vi "Parse Navigation Results.vi"(9 "Cycle Time":dbl, 10 "Targeting Data In":T1, 11 "Target Data":string) -> (2 "Targeting Data Out":T1)   [LabVIEW 2017, in "VisionHW.lvlib"]
uses:
  VisionHW.lvlib
  TypeDef/CLUST_Targeting Data.ctl
  TypeDef/CLUST_Cube Data.ctl
  TypeDef/CLUST_Road Navigation Data.ctl
  <vilib>/regexp/Match Regular Expression.xnode
panel:
  out "after substring":string
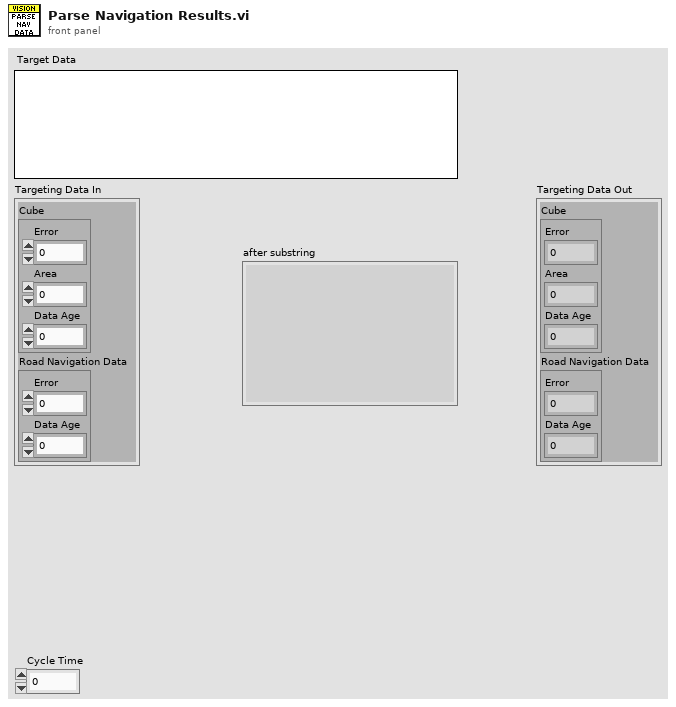
[diagram p1: front panel]
types:
  T1 = typedef "VisionHW.lvlib/CLUST_Targeting Data.ctl" = cluster{"Cube ":T2, "Road Navigation Data":T3}
  T2 = typedef "VisionHW.lvlib/CLUST_Cube Data.ctl" = cluster{"Error":dbl, "Area":dbl, "Data Age":dbl}
  T3 = typedef "VisionHW.lvlib/CLUST_Road Navigation Data.ctl" = cluster{"Error":i32, "Data Age":dbl}
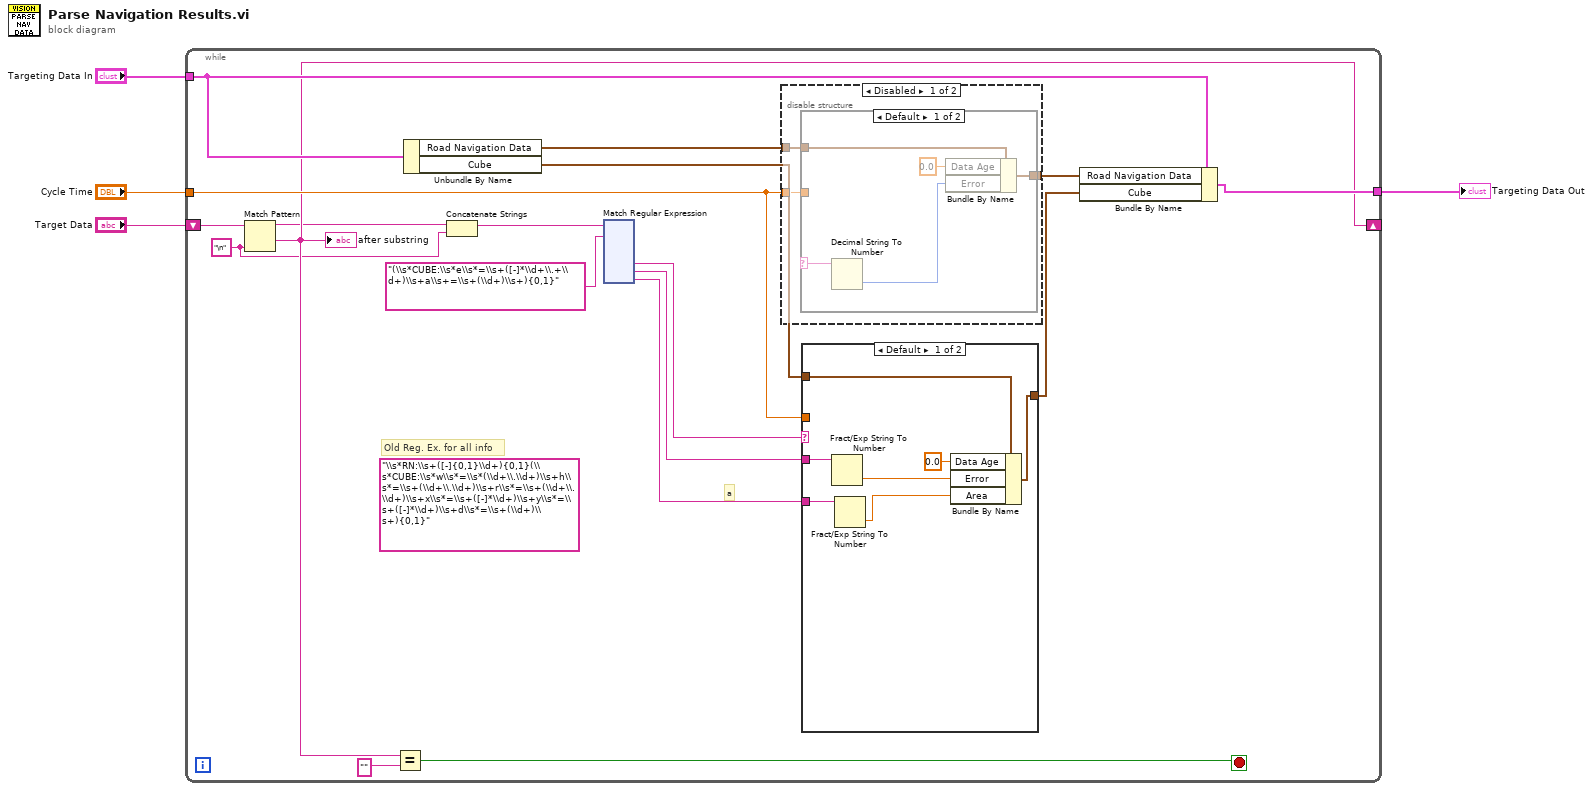
[diagram p0: block diagram]
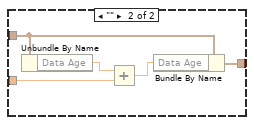
[diagram p2: hidden frame]
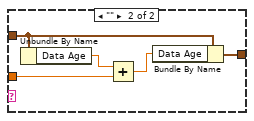
[diagram p4: hidden frame]
diagram:
  n1 = while {
    tunnel: "Cycle Time" -> [w19]
    tunnel: "Targeting Data In" -> [w17]
    tunnel: [w13] -> w2
    shift-right: [w11] -> _
    shift-left: "Target Data" -> [w12]
    stop <- w14 stop-if-true
    (unwired) "\\s*RN:\\s+([-]{0,1}\\d+){0,1}(\\s*CUBE:\\s*w\\s*=\\s*(\\d+\\.\\d+)\\s+h\\s*=\\s+(\\d+\\.\\d+)\\s+r\\s*=\\s+(\\d+\\.\\d+)\\s+x\\s*=\\s+([-]*\\d+)\\s+y\\s*=\\s+([-]*\\d+)\\s+d\\s*=\\s+(\\d+)\\s+){0,1}" ("regular expression")
    w9 = "\n" ("delimiter (Tab)")
    # "a"
    # "Old Reg. Ex. for all info"
    n2 = Match Pattern(string=w12, regular expression=w9) -> (before substring=w10:string, after substring=w11:string)  [unwired: 1 in, 2 out]
    "after substring" <- w11
    n3 = Equal?(x=w11, y="") -> (x = y?=w14:bool)
    n4 = Unbundle By Name(w17) -> ("Road Navigation Data"=w21:T3, "Cube"=w20:T2)
    n5 = Concatenate Strings(w10, w9) -> (w8:string)
    n6 = xnode "Match Regular Expression"("input string"=w8, "regular expression"="(\\s*CUBE:\\s*e\\s*=\\s+([-]*\\d+\\.+\\d+)\\s+a\\s+=\\s+(\\d+)\\s+){0,1}") -> ("submatch 1"=w7:string, "submatch 2"=w6:string, "submatch 3"=w5:string)  [unwired: 4 in, 5 out]
    n7 = disable-structure shown="Disabled" {
      disable-tunnel: w21 -> [w25 _]
      disable-tunnel: w19 -> [w24 _]
      disable-tunnel: [w23 _] -> w18
      frame Disabled {
        n8 = case shown="Default" {
          selector: _ -> [w30 _]
          tunnel: w25 -> [w29 w34]
          tunnel: [w26 w35] -> w23
          tunnel: w24 -> [_ w32]
          frame Default {
            n9 = Decimal String To Number(string=w30) -> (number=w28:i32)  [unwired: 2 in, 1 out]
            n10 = Bundle By Name(cluster=w29, "Data Age"=0.0, "Error"=w28) -> (w26:T3)
          }
          frame "" {
            n11 = Unbundle By Name(w34) -> ("Data Age"=w33:dbl)
            n12 = Add(x=w33, y=w32) -> (x+y=w31:dbl)
            n13 = Bundle By Name(cluster=w34, "Data Age"=w31) -> (w35:T3)
          }
        }
      }
      frame Enabled {
      }
    }
    n14 = case shown="Default" w7 {
      tunnel: w6 -> [w41 _]
      tunnel: w20 -> [w42 w47]
      tunnel: w19 -> [_ w43]
      tunnel: [w39 w46] -> w16
      tunnel: w5 -> [w37 _]
      frame Default {
        n15 = Fract/Exp String To Number(string=w41) -> (number=w38:dbl)  [unwired: 3 in, 1 out]
        n16 = Fract/Exp String To Number(string=w37) -> (number=w36:dbl)  [unwired: 3 in, 1 out]
        n17 = Bundle By Name(cluster=w42, "Data Age"=0.0, "Error"=w38, "Area"=w36) -> (w39:T2)
      }
      frame "" {
        n18 = Unbundle By Name(w47) -> ("Data Age"=w45:dbl)
        n19 = Add(x=w45, y=w43) -> (x+y=w44:dbl)
        n20 = Bundle By Name(cluster=w47, "Data Age"=w44) -> (w46:T2)
      }
    }
    n21 = Bundle By Name(cluster=w17, "Road Navigation Data"=w18, "Cube"=w16) -> (w13:T1)
  }
  "Targeting Data Out" <- w2
